vi "PKG_IMC_GetCapData.vi"(0 "handle":u32, 1 "lastNum":i32, 5 "rdnum":i32, 7 "pdata":i32, 9 "dataNum":i32, 12 "axis":i32) -> (3 "lastNum out":i32, 4 "handle out":u32, 6 "function return":i32, 8 "pdata out":i32, 10 "dataNum out":i32)   [LabVIEW 2011, in "IMC_Pkg4xxx.lvlib"]
doc: "PKG_IMC_GetCapData(IMC_HANDLE handle, int rdnum, long *pdata, int *dataNum, int *lastNum, int axis);"
uses:
  IMC_Pkg4xxx.lvlib
  IMC_Pkg4xxx.dll
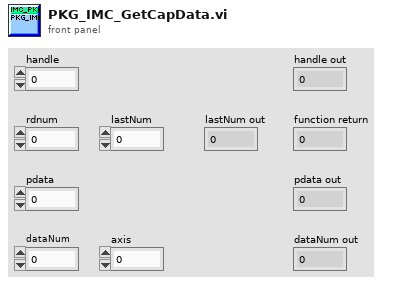
[diagram p1: front panel]
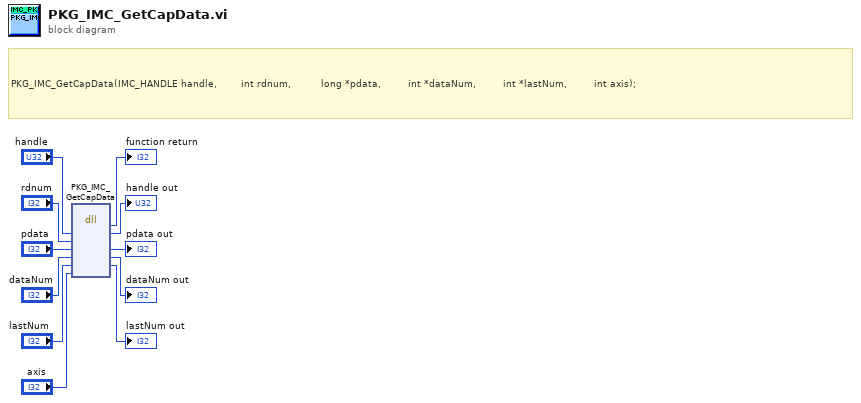
[diagram p0: block diagram]
diagram:
  # "PKG_IMC_GetCapData(IMC_HANDLE handle,  \t\t\t\t\t\tint rdnum, \t\t\t\t\t\t\t\t\tlong *pdata, \t\t\t\t\t\t\t\tint *dataNum, \t\t\t\t\t\t\t\tint *lastNum, \t\t\t\t\t\t\t\tint axis);"
  n1 = dll-call lib="PTH1mabs F光盘刻录\niMC MotionIMCNet_V4.0IMCAppincLabviewIMC_PKG4xxxIMC_PKG4xxx\nIMC_Pkg4xxx.*" fn="PKG_IMC_GetCapData"("handle"="handle", "rdnum"="rdnum", "pdata"="pdata", "dataNum"="dataNum", "lastNum"="lastNum", "axis"="axis") -> (→"function return":i32, "handle"=→"handle out":u32, "pdata"=→"pdata out":i32, "dataNum"=→"dataNum out":i32, "lastNum"=→"lastNum out":i32)  [unwired: 5 in, 2 out]
